vi "TemperatureWarnings.vi"() -> ()   [LabVIEW 2018]
doc: "Hannah Bussmann\n18.02.20\n\nThe VI is supposed to give a heatstroke Warning if the Current Temperature is greater or equal to the Max temperature. If the Current Temperature is less or equal to the Min Temperature there should be a freeze Warning. In every other case, there should be no Warning"
panel:
  out "Error Out":errorcluster
  in  "Error In":errorcluster
  out "Warning Text":string
  out "Warning?":bool
  in  "Min Temperature":dbl
  in  "Max Temperature":dbl
  in  "Current Temperature":dbl
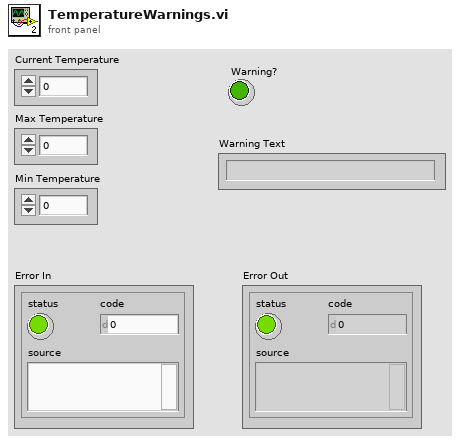
[diagram p1: front panel]
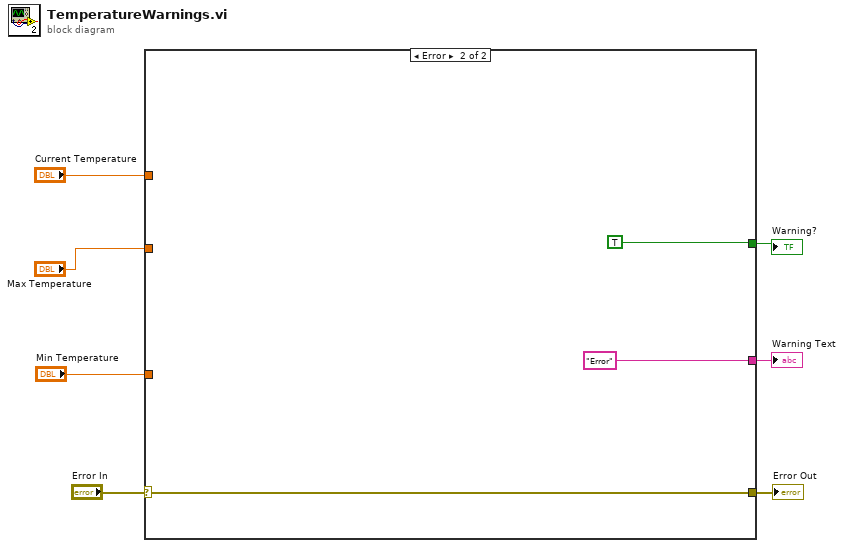
[diagram p0: block diagram]
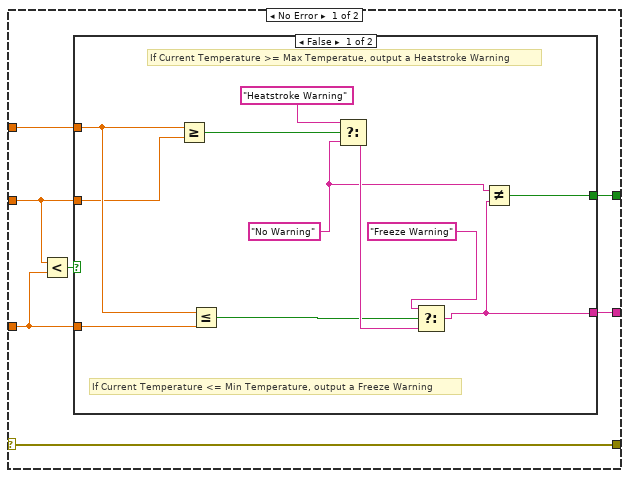
[diagram p2: hidden frame]
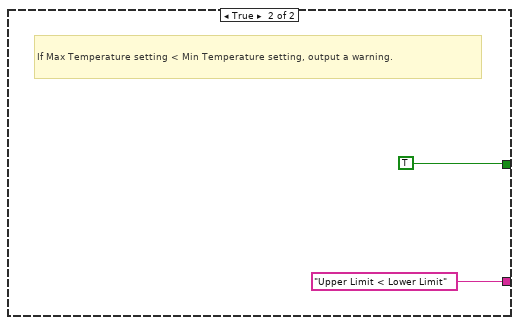
[diagram p3: hidden frame]
diagram:
  n1 = case shown="Error" "Error In" {
    selector: "Error In" -> [w10 w28]
    tunnel: "Current Temperature" -> [w14 _]
    tunnel: [w13 TRUE] -> w6
    tunnel: [w12 "Error"] -> w5
    tunnel: [w10 w28] -> w3
    tunnel: "Min Temperature" -> [w9 _]
    tunnel: "Max Temperature" -> [w8 _]
    frame No Error {
      n2 = Less?(x=w8, y=w9) -> (x < y?=w11:bool)
      n3 = case shown="False" w11 {
        tunnel: w14 -> [w25 _]
        tunnel: [w18 TRUE] -> w13
        tunnel: [w17 "Upper Limit < Lower Limit"] -> w12
        tunnel: w8 -> [w16 _]
        tunnel: w9 -> [w15 _]
        frame False {
          w19 = "No Warning"
          # "If Current Temperature <= Min Temperature, output a Freeze Warning"
          # "If Current Temperature >= Max Temperatue, output a Heatstroke Warning"
          n4 = Greater Or Equal?(x=w25, y=w16) -> (x >= y?=w21:bool)
          n5 = Less Or Equal?(x=w25, y=w15) -> (x <= y?=w20:bool)
          n6 = Select(t="Heatstroke Warning", s=w21, f=w19) -> (s? t:f=w22:string)
          n7 = Select(t="Freeze Warning", s=w20, f=w22) -> (s? t:f=w17:string)
          n8 = Not Equal?(x=w19, y=w17) -> (x != y?=w18:bool)
        }
        frame True {
          # "If Max Temperature setting < Min Temperature setting, output a warning."
        }
      }
    }
    frame Error {
    }
  }
  "Warning?" <- w6
  "Warning Text" <- w5
  "Error Out" <- w3
